vi "Set Property.vi"(10 "Ctl Ref":refnum<vi>, 11 "Template UIP In":refnum<class "PositionUIP.lvclass">) -> (0 "Error Out":errorcluster, 3 "Template UIP Out":refnum<class "PositionUIP.lvclass">)   [LabVIEW 2020, in "UIM.lvlib" / "PositionUIP.lvclass"]
doc: "Modify this method to implement functionality for applying the UIP data to the property from VI Server Control."
uses:
  PositionUIP.lvclass
  PositionUIP.lvclass/PositionUIP.ctl
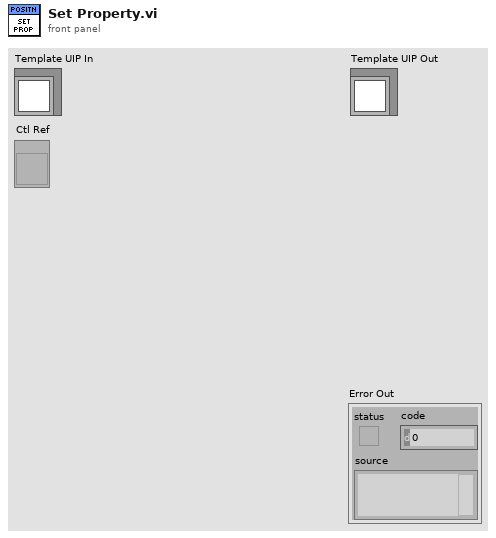
[diagram p1: front panel]
types:
  T1 = typedef "LVPositionTypeDef.ctl" = cluster{"Left":i32, "Top":i32}
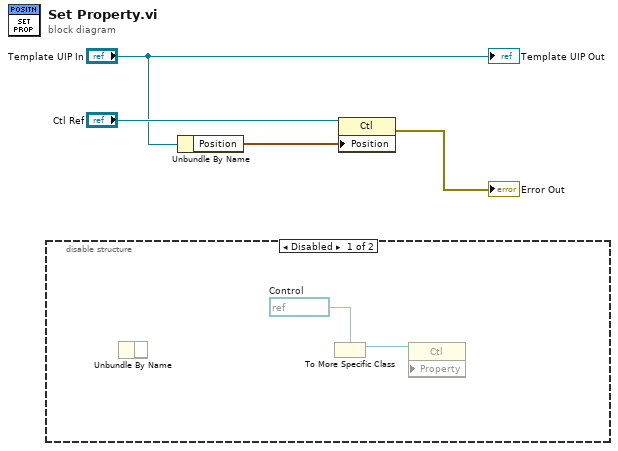
[diagram p0: block diagram]
diagram:
  n1 = disable-structure shown="Disabled" {
    frame Disabled {
      w6 = refnum<vi> refnum  # Control
      n2 = Unbundle By Name "Unbundle By Name"() -> ()  [unwired: 1 in, 1 out]
      n3 = To More Specific Class(target class=w6) -> (specific class reference=w5:refnum<vi>)  [unwired: 2 in, 1 out]
      n4 = property class="Ctl" props=[](reference=w5) -> ()  [unwired: 2 in, 2 out]
    }
    frame Enabled {
    }
  }
  n5 = Unbundle By Name("Template UIP In") -> ("Position"=w2:T1)
  n6 = property class="Ctl"(reference="Ctl Ref", "Position"=w2) -> (error out=→"Error Out":errorcluster)  [unwired: 1 in, 1 out]
  "Template UIP Out" <- "Template UIP In"
